vi "ParseDataa.vi"(9 "data out":string) -> (0 "Tank1":u16, 1 "Tank2":u16, 2 "Voltage":u16, 3 "Counter":u16)   [LabVIEW 2011]
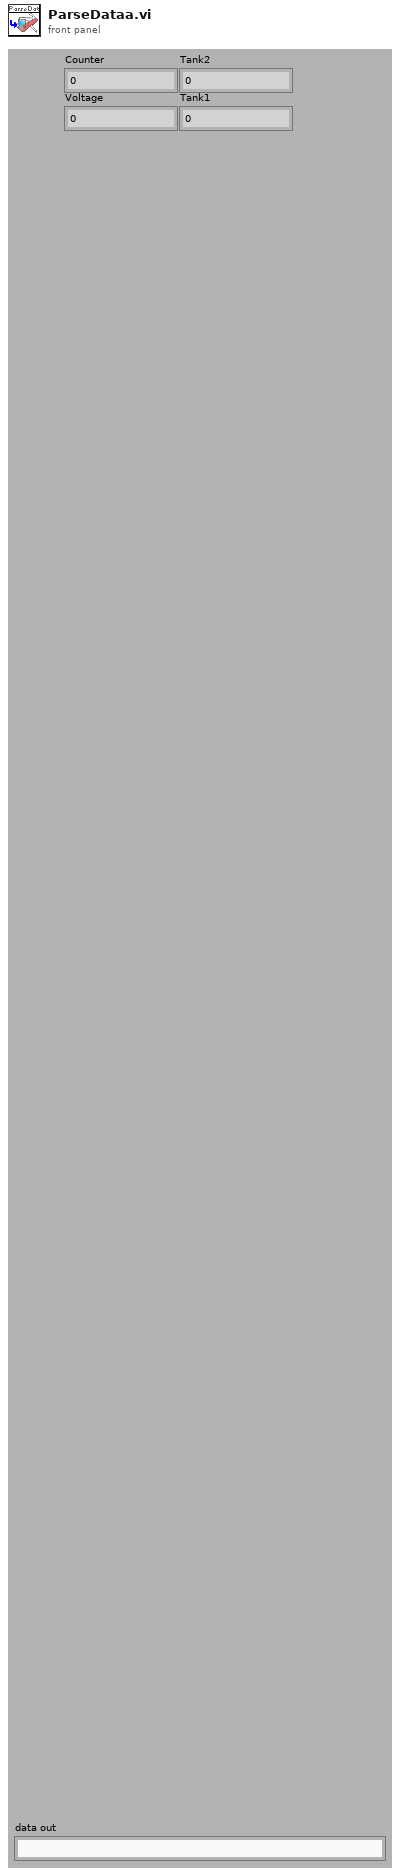
[diagram p1: front panel]
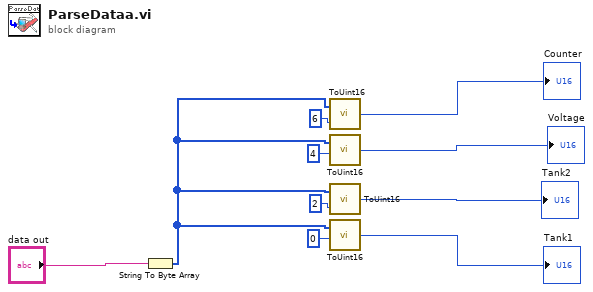
[diagram p0: block diagram]
diagram:
  n1 = String To Byte Array(string="data out") -> (unsigned byte array=w5:u8[])
  n2 = call "ToUint16.vi"("index"=6, "array"=w5) -> ("sp float"=→"Counter":u16)
  n3 = call "ToUint16.vi"("index"=4, "array"=w5) -> ("sp float"=→"Voltage":u16)
  n4 = call "ToUint16.vi"("index"=2, "array"=w5) -> ("sp float"=→"Tank2":u16)
  n5 = call "ToUint16.vi"("index"=0, "array"=w5) -> ("sp float"=→"Tank1":u16)
